vi "CalibrateFromImage.vi"() -> ()   [LabVIEW 2015]
uses:
  <vilib>/Utility/file.llb/Write Delimited Spreadsheet (DBL).vi
  <vilib>/vision/NI_Vision_Development_Module.lvlib
panel:
  out "Pixel to Real\n Conversion Factor":dbl
  out "Magnification":dbl
  in  "Line Real (mm)":dbl
  in  "Image to View":path
  in  "stop":bool
  out "Length or Distance (pixels)":sgl
  out "Image":T1(plugin-control)
  in  "Enum":enum16{"alpha 6000", "alpha nex-6"}(ring)
  # "Which Camera are you using?\n[Note: If you are using a new camera you will need to add it as an option \nin the code along with the sensor dimensions. Be careful taking the \nsensor dimensions straight from the manual because that is the entire \nsensor and the cameras tend to utilize less of the sensor for video.]"
  # "Input how long the line is in real life (mm)"
  # "Use only the line tool!"
  # "Press this button when you \nhave given a distance and \nyou are satisfied with your line."
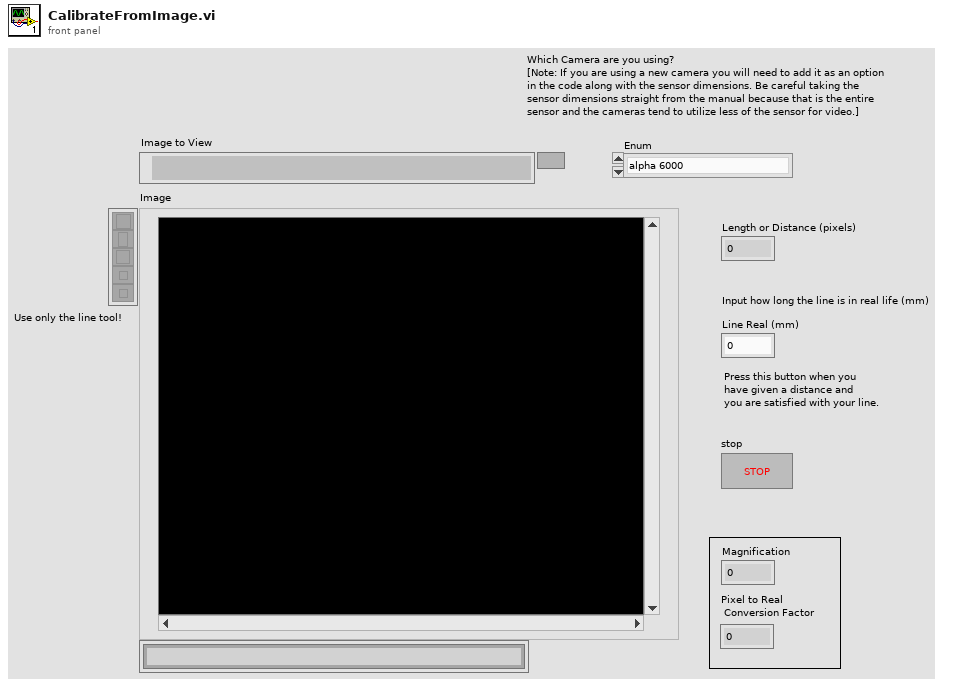
[diagram p1: front panel]
types:
  T1 = typedef "IMAQ Image.ctl" = refnum<image>
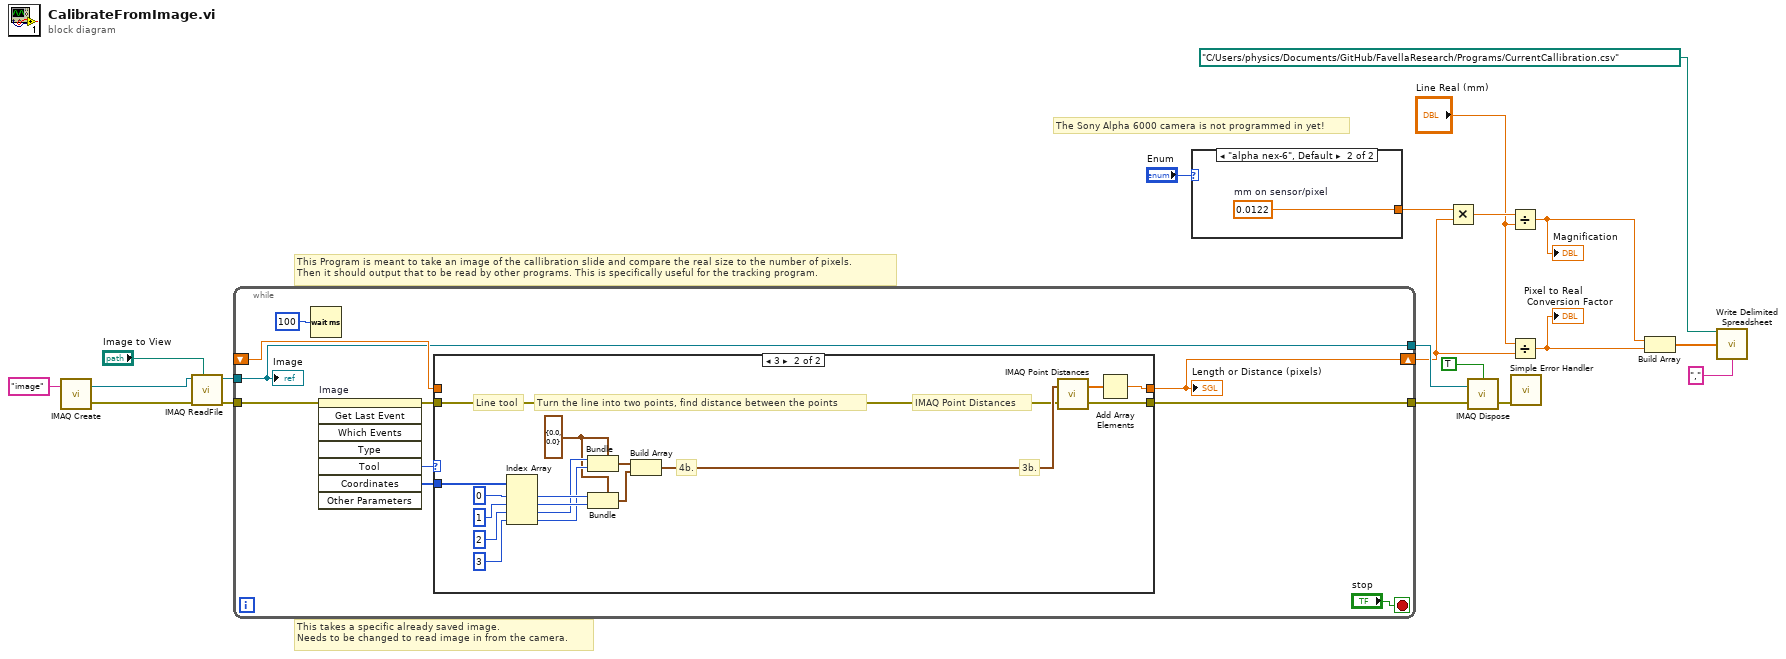
[diagram p0: block diagram]
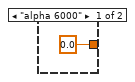
[diagram p3: hidden frame]
diagram:
  # "The Sony Alpha 6000 camera is not programmed in yet!"
  # "This takes a specific already saved image.\nNeeds to be changed to read image in from the camera."
  # "This Program is meant to take an image of the callibration slide and compare the real size to the number of pixels.\nThen it should output that to be read by other programs. This is specifically useful for the tracking program."
  n1 = call "IMAQ Create"("Image Name"="image") -> ("New Image"=w18:T1, "error out"=w19:errorcluster)  [unwired: 4 in]
  n2 = call "IMAQ ReadFile"("File Path"="Image to View", "error in (no error)"=w19, "Image"=w18) -> ("error out"=w16:errorcluster, "Image Out"=w17:T1)  [unwired: 4 in, 3 out]
  n3 = while {
    tunnel: w17 -> [w21]
    tunnel: [w30] -> w12
    tunnel: w16 -> [w24]
    shift-right: [w27] -> w6
    shift-left: _ -> [w26]
    tunnel: [w21] -> w13
    stop <- "stop" stop-if-true
    n4 = Wait (ms)(milliseconds to wait=u32 100) -> ()  [unwired: 1 out]
    n5 = invoke on="Image" class="ImageControl" method="Get Last Event"(error in=w24) -> (error out=w25:errorcluster, "Tool"=w23:i32, "Coordinates"=w22:i32[])  [unwired: 7 in, 5 out]
    n6 = case shown="3" w23 {
      tunnel: w22 -> [_ w38]
      tunnel: [w32 w34] -> w30
      tunnel: [w31 w35] -> w27
      tunnel: w25 -> [w32 w33]
      tunnel: w26 -> [w31 _]
      frame 0, Default {
        # "Do nothing if no new ROI is selected"
      }
      frame 3 {
        w37 = cluster{"X":sgl, "Y":sgl} {"X"=0.0, "Y"=0.0}
        # "Turn the line into two points, find distance between the points"
        # "Line tool"
        # "4b."
        # "3b."
        # "IMAQ Point Distances"
        n7 = Index Array(array=w38, index #1=0 ("index"), index #2=1 ("index"), index #3=2 ("index"), index #4=3 ("index")) -> (element #1=w45:i32, element #2=w44:i32, element #3=w43:i32, element #4=w42:i32)
        n8 = Bundle(cluster=w37, "X"=w43, "Y"=w42) -> (w41:cluster{"X":sgl, "Y":sgl})
        n9 = Bundle(cluster=w37, "X"=w45, "Y"=w44) -> (w40:cluster{"X":sgl, "Y":sgl})
        n10 = Build Array(w41, w40) -> (w39:cluster{"X":sgl, "Y":sgl}[])
        n11 = call "IMAQ Point Distances"("Points"=w39, "error in (no error)"=w33) -> ("Distances"=w36:sgl[], "error out"=w34:errorcluster)  [unwired: 3 in]
        n12 = Add Array Elements(numeric array=w36) -> (sum=w35:sgl)
      }
    }
    "Length or Distance (pixels)" <- w27
    "Image" <- w21
  }
  n13 = case shown="\"alpha nex-6\", Default" "Enum" {
    tunnel: [0.0 w51] -> w9
    frame "alpha 6000" {
    }
    frame "alpha nex-6", Default {
      w51 = 0.0122  # mm on sensor/pixel
    }
  }
  n14 = Multiply(x=w9, y=w6) -> (x*y=w8:dbl)
  n15 = call "IMAQ Dispose"("All Images? (No)"=TRUE, "Image"=w13, "error in (no error)"=w12) -> ("error out"=w10:errorcluster)  [unwired: 3 in]
  n16 = Divide(x=w8, y="Line Real (mm)") -> (x/y=w3:dbl)
  "Magnification" <- w3
  n17 = Divide(x="Line Real (mm)", y=w6) -> (x/y=w4:dbl)
  "Pixel to Real\n Conversion Factor" <- w4
  n18 = call <vilib>:"Simple Error Handler.vi"("error in (no error)"=w10) -> ()  [unwired: 4 in, 5 out]
  n19 = Build Array(w3, w4) -> (w1:dbl[])
  n20 = call-poly <vilib>:"Write Delimited Spreadsheet.vi"("file path (dialog if empty)"=path "C:/Users/physics/Documents/GitHub/FavellaResearch/Programs/CurrentCallibration.csv", "1D data"=w1, "delimiter (\\t)"=",") -> ()  [unwired: 11 in, 2 out]
